vi "TestModeUpdate.vi"(8 "error in (no error)":errorcluster, 11 "Update?":bool) -> (0 "error out":errorcluster, 3 "conf'":T1={"Test Mode"=enum."6.3.2 저온 작동/방치 시험", "ON time[ms]"=500.0, "OFF time[ms]"=10000.0, "1. 작동시간[분]"=10000.0, "2. 미작동시간[분]"=10000.0, "3. 작동시간[분]"=10000.0, "level[V]"=12.0, "duty"=20.0, "Freq"=1.0, "Voltage+[V]"=20.0, "Voltage-[V]"=-20.0, "Current+[A]"=5.0, "Current-[A]"=-5.0, "출력전압[V]"=0.0, "출력전류[A]"=0.0, "OVP Level"=0.0, "OCP Level"=0.0, "Time Div"=0, "Record Len"=4, "방전 기준[V]"=0.0, "Repeate (Each Ch)"=1, "Cycle[N]"=1, "작동간격[분]"=10000.0, "TrigPos[%]"=0.0, "시험시간[분]"=10000.0} {"시험시간[분]" min=1.0; "작동간격[분]" min=1.0; "3. 작동시간[분]" min=1.0; "2. 미작동시간[분]" min=1.0; "1. 작동시간[분]" min=1.0; "Time Div" items=["10m", "20ms", "50ms", "100ms", "200ms", "500ms", "1s", "2s", "5s", "10s", "20s", "30s", "1min", "2min", "5min"]; "OFF time[ms]" min=10000.0 max=1000000.0; "Current-[A]" min=-20.0 max=20.0 step=0.001; "Voltage-[V]" min=-115.0 max=115.0 step=0.01; "Current+[A]" min=0.0 max=60.0 step=0.01; "Voltage+[V]" min=0.0 max=120.0 step=0.1; "OCP Level" format="%#_13g"; "OVP Level" format="%#_13g"; "Record Len" items=["10k", "25k", "50k", "100k", "250k", "500k", "1M", "2.5M", "5M", "10M", "25M", "50M", "100M", "250M", "500M", "1G", "2G", "4G", "5G", "10G", "20G", "50G"]; "ON time[ms]" min=50.0 max=2000000.0})   [LabVIEW 2019]
uses:
  Durability/Capacitor/cap_config.ctl
  _ctrl/rw.ctl
  Durability/common/Global 1.vi
panel:
  out "Array":string[](array[string])
  # "제어단 전압"
  # "출력단 전원"
  # "DL950"
  # "Discharge"
  # "Test Cycle"
  # "작동 설정"
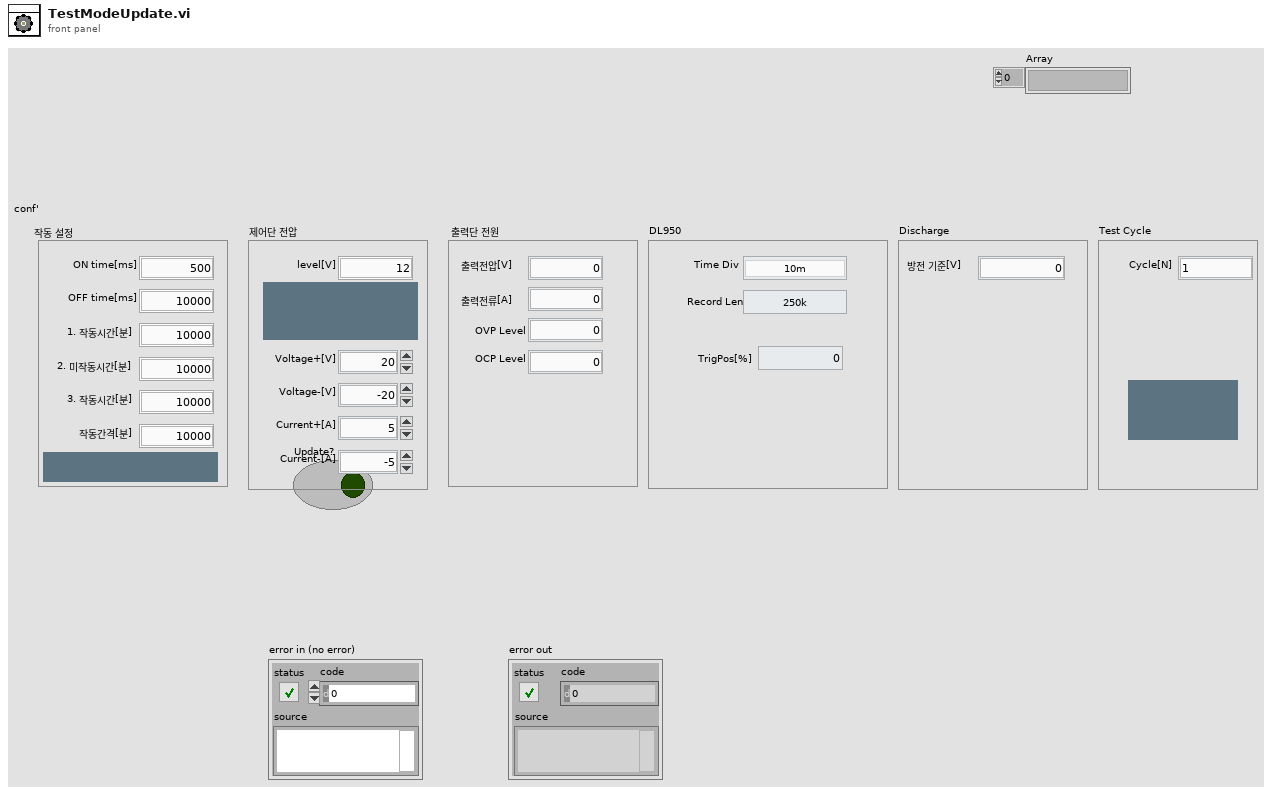
[diagram p1: front panel]
types:
  T1 = typedef "cap_config.ctl" = cluster{"Test Mode":T2, "ON time[ms]":dbl, "OFF time[ms]":dbl, "1. 작동시간[분]":dbl, "2. 미작동시간[분]":dbl, "3. 작동시간[분]":dbl, "level[V]":dbl, "duty":dbl, "Freq":dbl, "Voltage+[V]":dbl, "Voltage-[V]":dbl, "Current+[A]":dbl, "Current-[A]":dbl, "출력전압[V]":dbl, "출력전류[A]":dbl, "OVP Level":dbl, "OCP Level":dbl, "Time Div":u16, "Record Len":i32, "방전 기준[V]":dbl, "Repeate (Each Ch)":u32, "Cycle[N]":u32, "작동간격[분]":dbl, "TrigPos[%]":dbl, "시험시간[분]":dbl}
  T2 = typedef "시험모드선택.ctl" = enum16{"6.3.1 온도방치 시험", "6.3.2 저온 작동/방치 시험", "6.3.3 고온 작동/방치 시험", "6.3.4 온도 싸이클 시험", "6.3.6 온습도 싸이클 시험", "6.3.7 고온고습 방치", "6.3.8 결로 시험", "6.3.9 빙결시험", "6.3.10 공진", "6.3.11.1 작동가진", "6.3.11.2 비작동 가진 ", "6.3.12 충격시험"}
  T3 = typedef "rw.ctl" = enum16{"read", "write"}
  T4 = typedef "ref_all.ctl" = cluster{"BP4610 Config":refnum<vi>, "DSP1950 Config":refnum<vi>, "2470-config":refnum<vi>, "cDAQ 9269 AO config":refnum<vi>, "cDAQ 9221 Config":refnum<vi>, "cDAQ-9467 Config":refnum<vi>, "Waveform":refnum<vi>, "DL950 wfm":refnum<vi>, "AI Graph":refnum<vi>, "AO_Wave-config":refnum<vi>, "DL950 items":refnum<vi>, "Volt":refnum<vi>, "Current":refnum<vi>, "AO_Level":refnum<vi>, "RC-Test Judgement ":refnum<vi>, "Log path":refnum<vi>, "시험명":refnum<vi>, "file renew[Hr]":refnum<vi>, "Breakdown-Spec":refnum<vi>, "paste":refnum<vi>, "copy":refnum<vi>, "DL950_config":refnum<vi>, "종료시간":refnum<vi>, "경과시간":refnum<vi>, "Apply":refnum<vi>, "DSP Config LV ":refnum<vi>, "Testconfig":refnum<vi>}
  T5 = typedef "Test Mode.ctl" = enum32{"저항부하", "캐패시터부하", "B수명 - 1", "B수명 - 2", "B수명 - 3", "저전압모드 동작검사", "저전압모드 접촉저항", "고전압모드 동작검사"}
  T6 = enum32{"6.3.2 저온 작동/방치 시험", "6.3.3 고온 작동/방치 시험", "6.3.4 온도 싸이클 시험", "6.3.6 온습도 싸이클 시험", "6.3.8 결로 시험", "6.3.9 빙결 시험"}
  T7 = enum8{"Enabled", "Disabled", "Disabled and Grayed Out"}[]
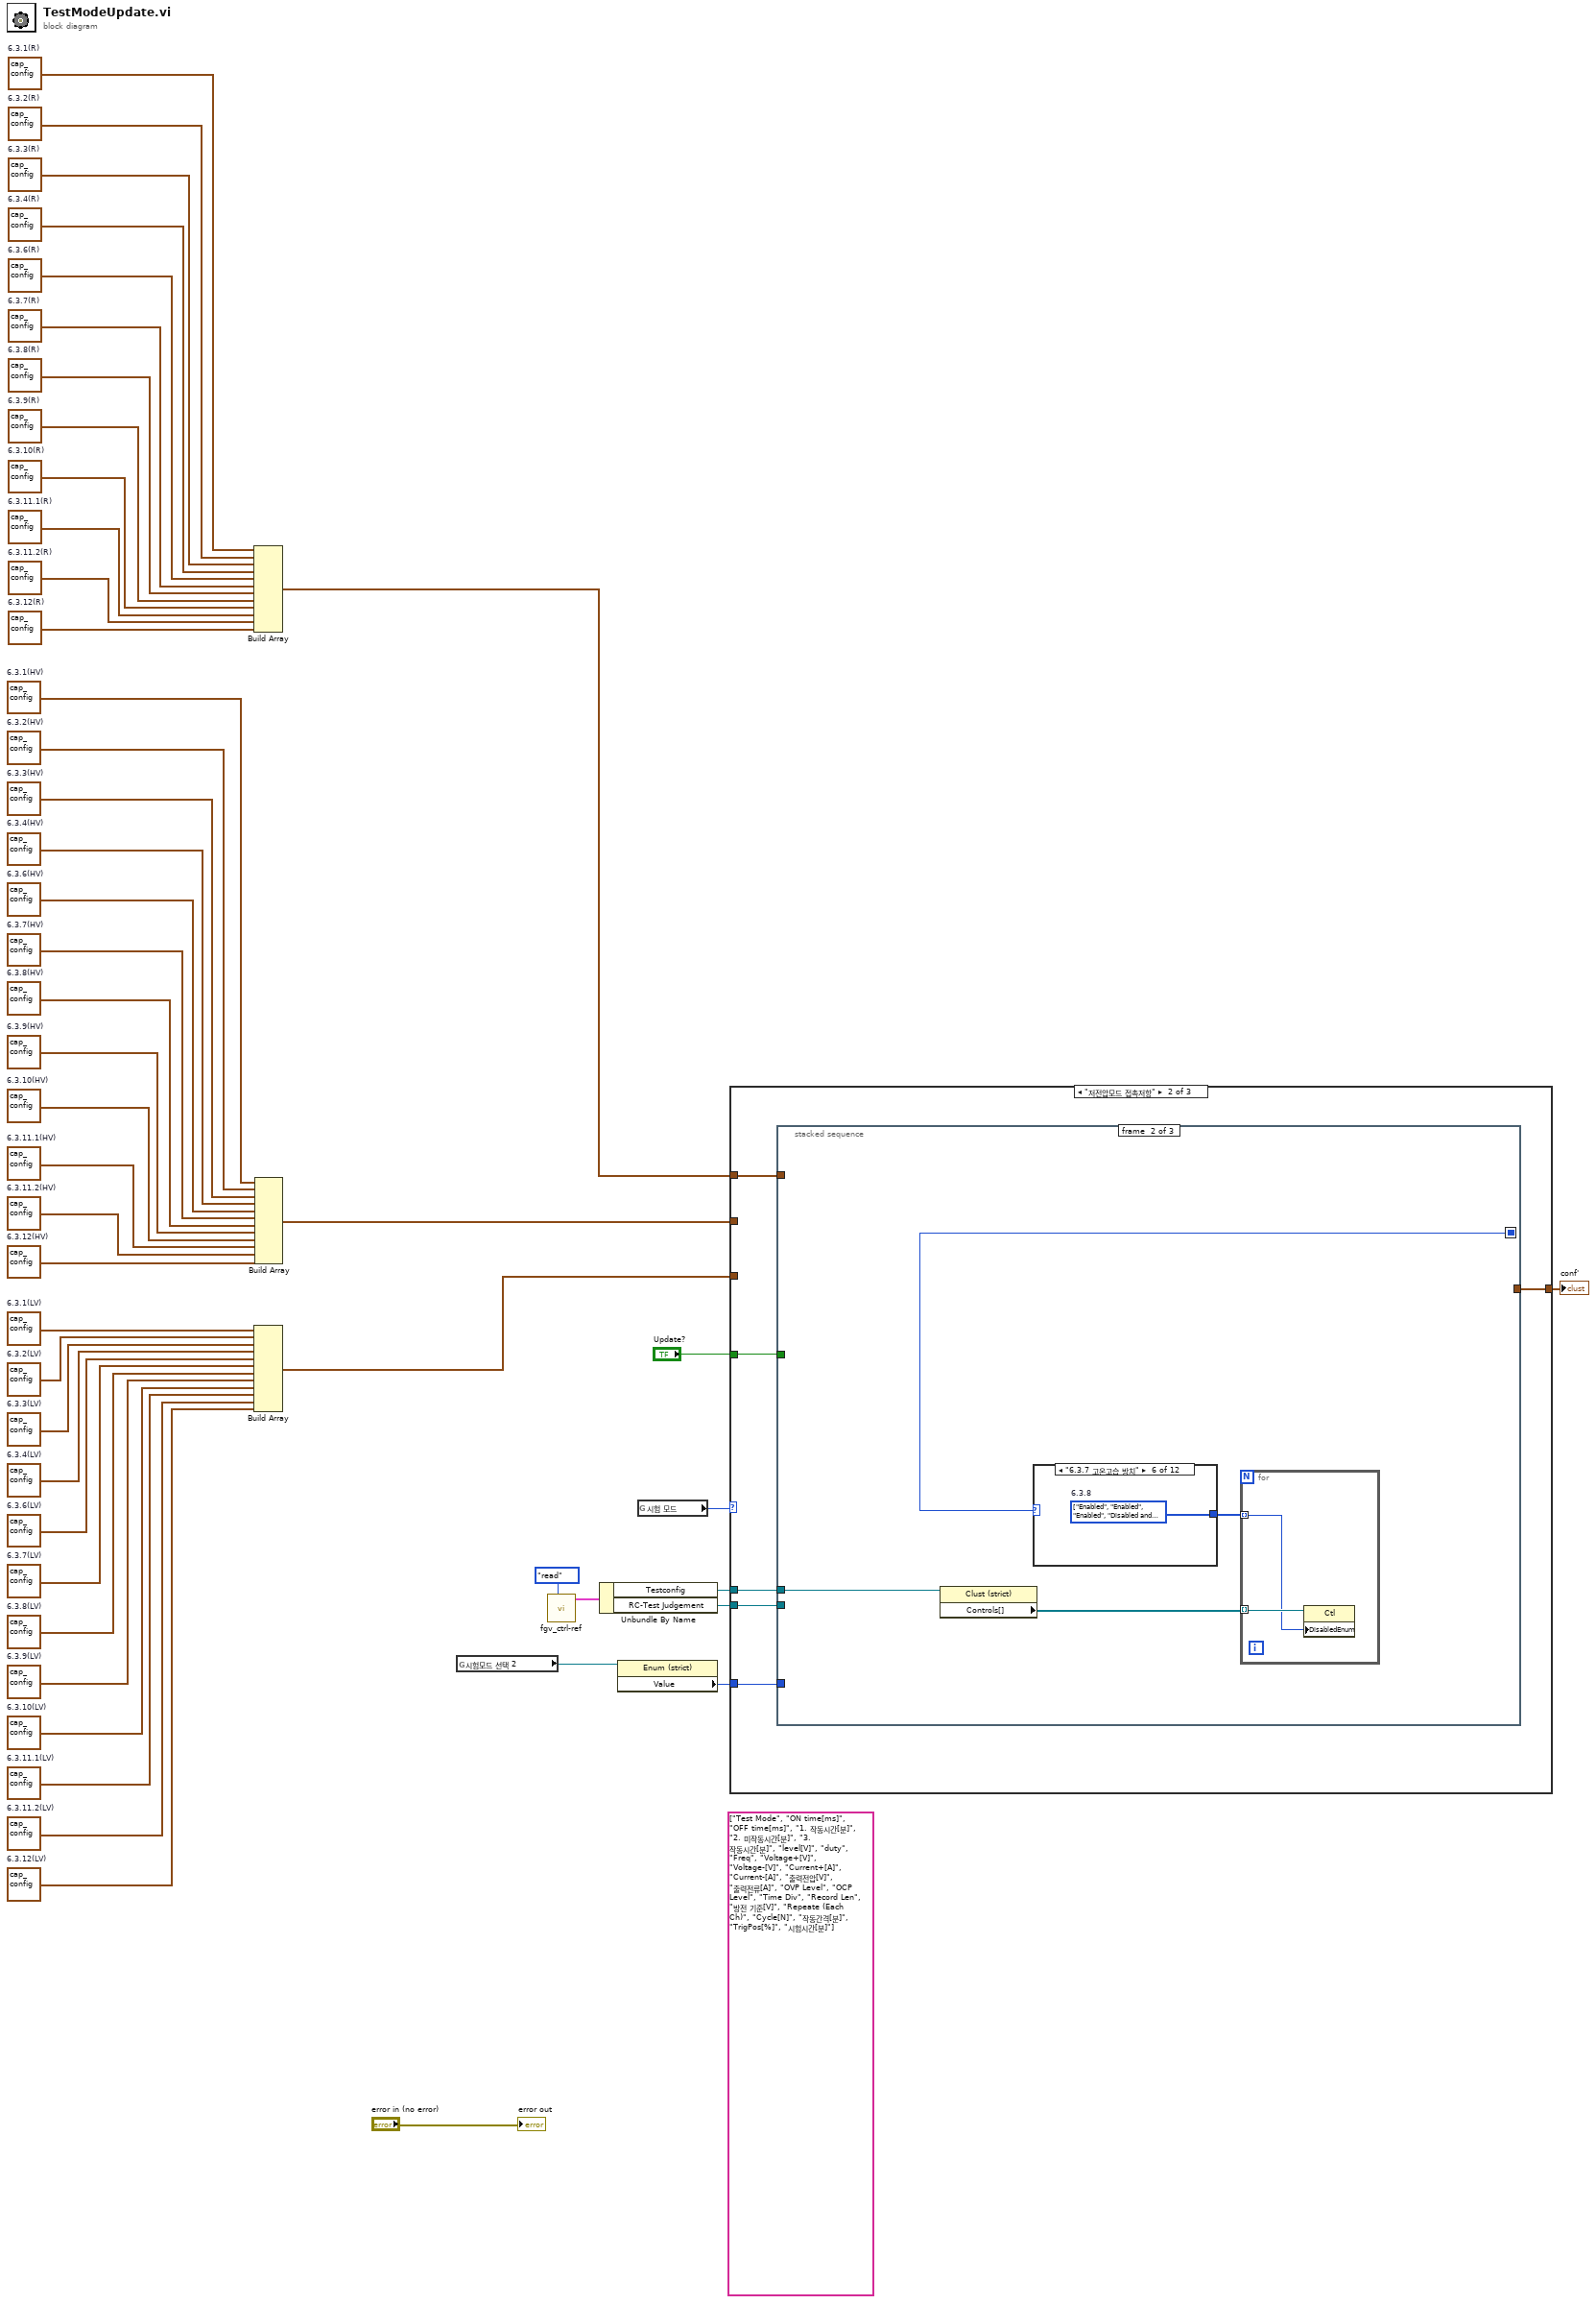
[diagram p0: block diagram]
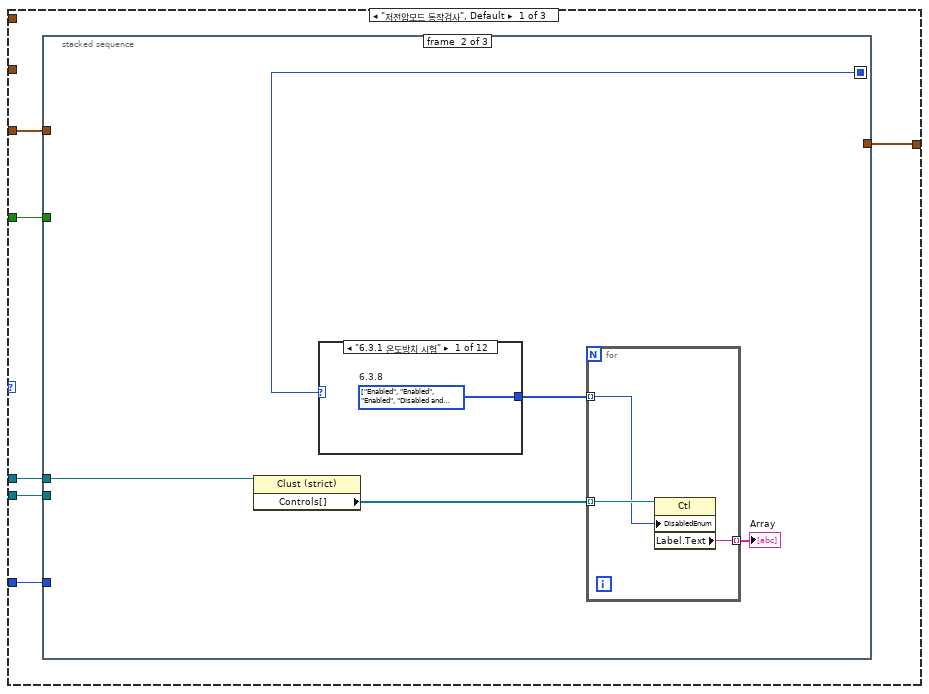
[diagram p2: hidden frame]
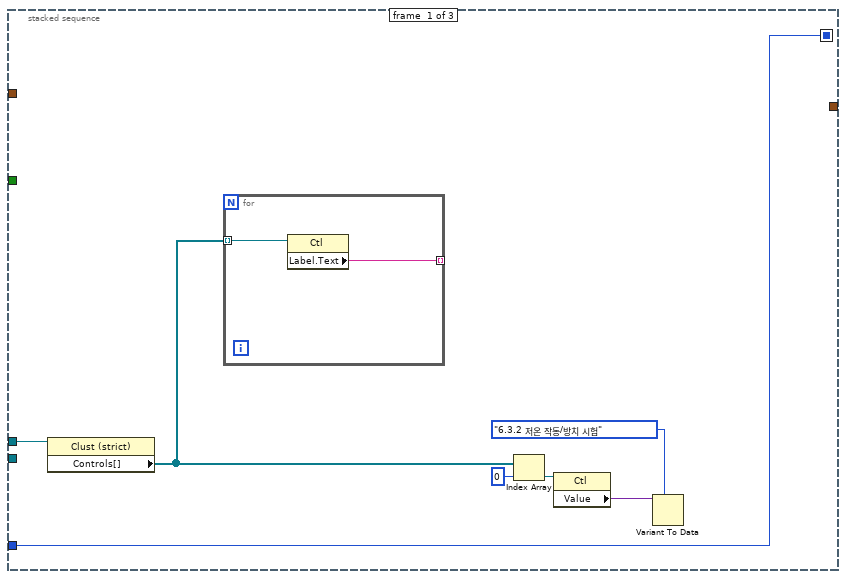
[diagram p3: hidden frame]
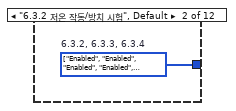
[diagram p4: hidden frame]
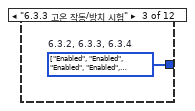
[diagram p5: hidden frame]
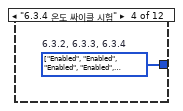
[diagram p6: hidden frame]
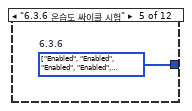
[diagram p7: hidden frame]
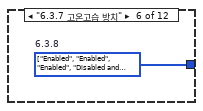
[diagram p8: hidden frame]
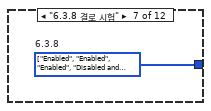
[diagram p9: hidden frame]
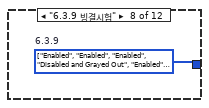
[diagram p10: hidden frame]
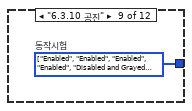
[diagram p11: hidden frame]
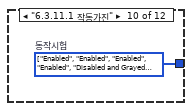
[diagram p12: hidden frame]
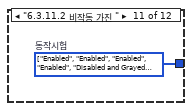
[diagram p13: hidden frame]
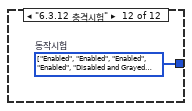
[diagram p14: hidden frame]
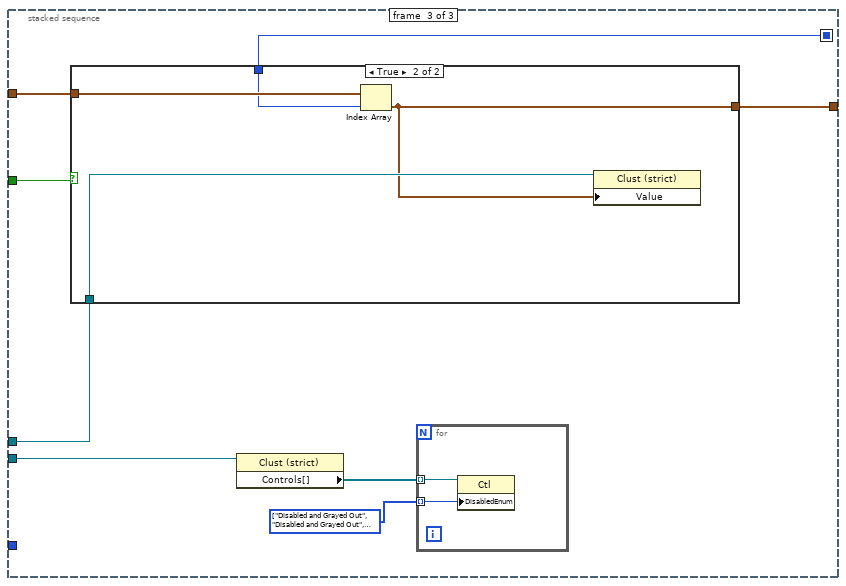
[diagram p15: hidden frame]
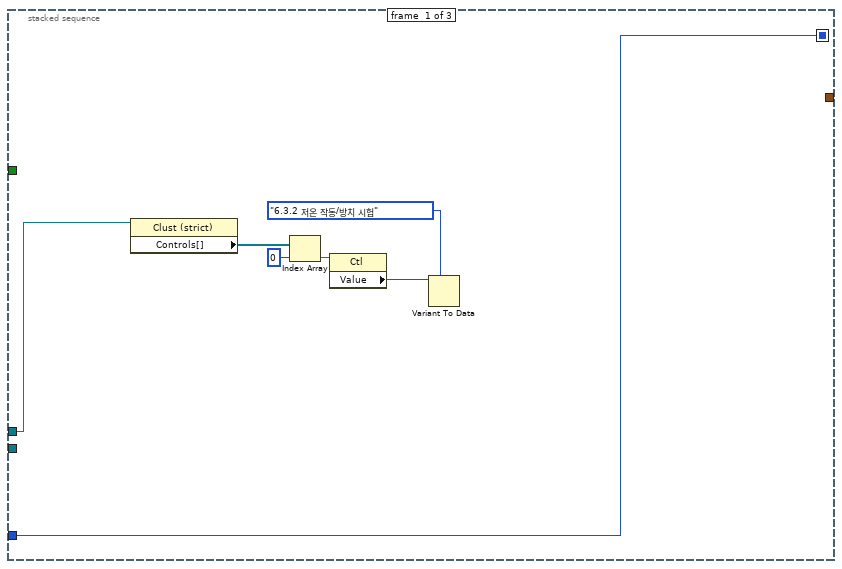
[diagram p17: hidden frame]
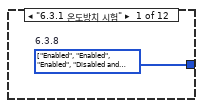
[diagram p18: hidden frame]
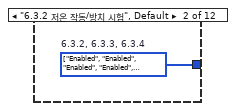
[diagram p19: hidden frame]
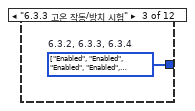
[diagram p20: hidden frame]
diagram:
  (unwired) string[] ["Test Mode", "ON time[ms]", "OFF time[ms]", "1. 작동시간[분]", "2. 미작동시간[분]", "3. 작동시간[분]", "level[V]", "duty", "Freq", "Voltage+[V]", "Voltage-[V]", "Current+[A]", "Current-[A]", "출력전압[V]", "출력전류[A]", "OVP Level", "OCP Level", "Time Div", "Record Len", "방전 기준[V]", "Repeate (Each Ch)", "Cycle[N]", "작동간격[분]", "TrigPos[%]", "시험시간[분]"] ("Array")
  w2 = T1 {"Test Mode"=enum."6.3.11.2 비작동 가진 ", "ON time[ms]"=200.0, "OFF time[ms]"=10000.0, "1. 작동시간[분]"=5.0, "2. 미작동시간[분]"=0.0, "3. 작동시간[분]"=0.0, "level[V]"=12.0, "duty"=100.0, "Freq"=1.0, "Voltage+[V]"=20.0, "Voltage-[V]"=-20.0, "Current+[A]"=5.0, "Current-[A]"=-5.0, "출력전압[V]"=12.0, "출력전류[A]"=2.0, "OVP Level"=20.0, "OCP Level"=5.0, "Time Div"=2, "Record Len"=5, "방전 기준[V]"=0.0, "Repeate (Each Ch)"=1, "Cycle[N]"=1, "작동간격[분]"=0.0, "TrigPos[%]"=10.0, "시험시간[분]"=0.0}  # 6.3.11.2(LV)
  w4 = T1 {"Test Mode"=enum."6.3.10 공진", "ON time[ms]"=200.0, "OFF time[ms]"=10000.0, "1. 작동시간[분]"=20.0, "2. 미작동시간[분]"=0.0, "3. 작동시간[분]"=0.0, "level[V]"=12.0, "duty"=100.0, "Freq"=1.0, "Voltage+[V]"=20.0, "Voltage-[V]"=-20.0, "Current+[A]"=5.0, "Current-[A]"=-5.0, "출력전압[V]"=12.0, "출력전류[A]"=2.0, "OVP Level"=20.0, "OCP Level"=5.0, "Time Div"=2, "Record Len"=5, "방전 기준[V]"=0.0, "Repeate (Each Ch)"=1, "Cycle[N]"=1, "작동간격[분]"=0.0, "TrigPos[%]"=10.0, "시험시간[분]"=0.0}  # 6.3.10(LV)
  w6 = T1 {"Test Mode"=enum."6.3.11.2 비작동 가진 ", "ON time[ms]"=200.0, "OFF time[ms]"=10000.0, "1. 작동시간[분]"=5.0, "2. 미작동시간[분]"=0.0, "3. 작동시간[분]"=0.0, "level[V]"=12.0, "duty"=100.0, "Freq"=1.0, "Voltage+[V]"=20.0, "Voltage-[V]"=-20.0, "Current+[A]"=5.0, "Current-[A]"=-5.0, "출력전압[V]"=450.0, "출력전류[A]"=30.0, "OVP Level"=1000.0, "OCP Level"=50.0, "Time Div"=2, "Record Len"=5, "방전 기준[V]"=1.0, "Repeate (Each Ch)"=1, "Cycle[N]"=1, "작동간격[분]"=0.0, "TrigPos[%]"=10.0, "시험시간[분]"=0.0}  # 6.3.11.2(HV)
  w8 = T1 {"Test Mode"=enum."6.3.10 공진", "ON time[ms]"=200.0, "OFF time[ms]"=10000.0, "1. 작동시간[분]"=20.0, "2. 미작동시간[분]"=0.0, "3. 작동시간[분]"=0.0, "level[V]"=12.0, "duty"=100.0, "Freq"=1.0, "Voltage+[V]"=20.0, "Voltage-[V]"=-20.0, "Current+[A]"=5.0, "Current-[A]"=-5.0, "출력전압[V]"=450.0, "출력전류[A]"=30.0, "OVP Level"=1000.0, "OCP Level"=50.0, "Time Div"=2, "Record Len"=5, "방전 기준[V]"=1.0, "Repeate (Each Ch)"=1, "Cycle[N]"=1, "작동간격[분]"=0.0, "TrigPos[%]"=10.0, "시험시간[분]"=0.0}  # 6.3.10(HV)
  w12 = T1 {"Test Mode"=enum."6.3.10 공진", "ON time[ms]"=200.0, "OFF time[ms]"=10000.0, "1. 작동시간[분]"=20.0, "2. 미작동시간[분]"=0.0, "3. 작동시간[분]"=0.0, "level[V]"=12.0, "duty"=100.0, "Freq"=1.0, "Voltage+[V]"=20.0, "Voltage-[V]"=-20.0, "Current+[A]"=5.0, "Current-[A]"=-5.0, "출력전압[V]"=12.0, "출력전류[A]"=1.0, "OVP Level"=20.0, "OCP Level"=5.0, "Time Div"=2, "Record Len"=5, "방전 기준[V]"=0.0, "Repeate (Each Ch)"=1, "Cycle[N]"=1, "작동간격[분]"=1.0, "TrigPos[%]"=10.0, "시험시간[분]"=1.0}  # 6.3.10(R)
  w10 = T1 {"Test Mode"=enum."6.3.11.2 비작동 가진 ", "ON time[ms]"=200.0, "OFF time[ms]"=10000.0, "1. 작동시간[분]"=5.0, "2. 미작동시간[분]"=0.0, "3. 작동시간[분]"=0.0, "level[V]"=12.0, "duty"=100.0, "Freq"=1.0, "Voltage+[V]"=20.0, "Voltage-[V]"=-20.0, "Current+[A]"=5.0, "Current-[A]"=-5.0, "출력전압[V]"=12.0, "출력전류[A]"=1.0, "OVP Level"=20.0, "OCP Level"=5.0, "Time Div"=2, "Record Len"=5, "방전 기준[V]"=0.0, "Repeate (Each Ch)"=1, "Cycle[N]"=1, "작동간격[분]"=1.0, "TrigPos[%]"=10.0, "시험시간[분]"=1.0}  # 6.3.11.2(R)
  w30 = T1 {"Test Mode"=enum."6.3.8 결로 시험", "ON time[ms]"=200.0, "OFF time[ms]"=10000.0, "1. 작동시간[분]"=1.0, "2. 미작동시간[분]"=120.0, "3. 작동시간[분]"=60.0, "level[V]"=12.0, "duty"=100.0, "Freq"=1.0, "Voltage+[V]"=20.0, "Voltage-[V]"=-20.0, "Current+[A]"=5.0, "Current-[A]"=-5.0, "출력전압[V]"=12.0, "출력전류[A]"=1.0, "OVP Level"=20.0, "OCP Level"=5.0, "Time Div"=2, "Record Len"=5, "방전 기준[V]"=0.0, "Repeate (Each Ch)"=1, "Cycle[N]"=2, "작동간격[분]"=10.0, "TrigPos[%]"=10.0, "시험시간[분]"=60.0}  # 6.3.8(R)
  w3 = T1 {"Test Mode"=enum."6.3.11.1 작동가진", "ON time[ms]"=200.0, "OFF time[ms]"=10000.0, "1. 작동시간[분]"=1440.0, "2. 미작동시간[분]"=0.0, "3. 작동시간[분]"=0.0, "level[V]"=12.0, "duty"=100.0, "Freq"=1.0, "Voltage+[V]"=20.0, "Voltage-[V]"=-20.0, "Current+[A]"=5.0, "Current-[A]"=-5.0, "출력전압[V]"=12.0, "출력전류[A]"=2.0, "OVP Level"=20.0, "OCP Level"=5.0, "Time Div"=2, "Record Len"=5, "방전 기준[V]"=0.0, "Repeate (Each Ch)"=1, "Cycle[N]"=1, "작동간격[분]"=0.0, "TrigPos[%]"=10.0, "시험시간[분]"=0.0}  # 6.3.11.1(LV)
  w15 = T1 {"Test Mode"=enum."6.3.7 고온고습 방치", "ON time[ms]"=200.0, "OFF time[ms]"=10000.0, "1. 작동시간[분]"=0.0, "2. 미작동시간[분]"=10080.0, "3. 작동시간[분]"=10080.0, "level[V]"=12.0, "duty"=100.0, "Freq"=1.0, "Voltage+[V]"=20.0, "Voltage-[V]"=-20.0, "Current+[A]"=5.0, "Current-[A]"=-5.0, "출력전압[V]"=12.0, "출력전류[A]"=2.0, "OVP Level"=20.0, "OCP Level"=5.0, "Time Div"=2, "Record Len"=5, "방전 기준[V]"=0.0, "Repeate (Each Ch)"=1, "Cycle[N]"=1, "작동간격[분]"=0.0, "TrigPos[%]"=10.0, "시험시간[분]"=0.0}  # 6.3.7(LV)
  w20 = T1 {"Test Mode"=enum."6.3.1 온도방치 시험", "ON time[ms]"=200.0, "OFF time[ms]"=10000.0, "1. 작동시간[분]"=0.0, "2. 미작동시간[분]"=720.0, "3. 작동시간[분]"=720.0, "level[V]"=12.0, "duty"=100.0, "Freq"=1.0, "Voltage+[V]"=20.0, "Voltage-[V]"=-20.0, "Current+[A]"=5.0, "Current-[A]"=-5.0, "출력전압[V]"=12.0, "출력전류[A]"=2.0, "OVP Level"=20.0, "OCP Level"=5.0, "Time Div"=2, "Record Len"=5, "방전 기준[V]"=0.0, "Repeate (Each Ch)"=1, "Cycle[N]"=1, "작동간격[분]"=0.0, "TrigPos[%]"=10.0, "시험시간[분]"=0.0}  # 6.3.1(LV)
  w7 = T1 {"Test Mode"=enum."6.3.11.1 작동가진", "ON time[ms]"=200.0, "OFF time[ms]"=10000.0, "1. 작동시간[분]"=1440.0, "2. 미작동시간[분]"=0.0, "3. 작동시간[분]"=0.0, "level[V]"=12.0, "duty"=100.0, "Freq"=1.0, "Voltage+[V]"=20.0, "Voltage-[V]"=-20.0, "Current+[A]"=5.0, "Current-[A]"=-5.0, "출력전압[V]"=450.0, "출력전류[A]"=30.0, "OVP Level"=1000.0, "OCP Level"=50.0, "Time Div"=2, "Record Len"=5, "방전 기준[V]"=1.0, "Repeate (Each Ch)"=1, "Cycle[N]"=1, "작동간격[분]"=0.0, "TrigPos[%]"=10.0, "시험시간[분]"=0.0}  # 6.3.11.1(HV)
  w23 = T1 {"Test Mode"=enum."6.3.7 고온고습 방치", "ON time[ms]"=200.0, "OFF time[ms]"=10000.0, "1. 작동시간[분]"=0.0, "2. 미작동시간[분]"=10080.0, "3. 작동시간[분]"=10080.0, "level[V]"=12.0, "duty"=100.0, "Freq"=1.0, "Voltage+[V]"=20.0, "Voltage-[V]"=-20.0, "Current+[A]"=5.0, "Current-[A]"=-5.0, "출력전압[V]"=450.0, "출력전류[A]"=30.0, "OVP Level"=1000.0, "OCP Level"=50.0, "Time Div"=2, "Record Len"=5, "방전 기준[V]"=1.0, "Repeate (Each Ch)"=1, "Cycle[N]"=1, "작동간격[분]"=0.0, "TrigPos[%]"=10.0, "시험시간[분]"=0.0}  # 6.3.7(HV)
  w28 = T1 {"Test Mode"=enum."6.3.1 온도방치 시험", "ON time[ms]"=200.0, "OFF time[ms]"=10000.0, "1. 작동시간[분]"=0.0, "2. 미작동시간[분]"=720.0, "3. 작동시간[분]"=720.0, "level[V]"=12.0, "duty"=100.0, "Freq"=1.0, "Voltage+[V]"=20.0, "Voltage-[V]"=-20.0, "Current+[A]"=5.0, "Current-[A]"=-5.0, "출력전압[V]"=450.0, "출력전류[A]"=30.0, "OVP Level"=1000.0, "OCP Level"=50.0, "Time Div"=2, "Record Len"=5, "방전 기준[V]"=1.0, "Repeate (Each Ch)"=1, "Cycle[N]"=1, "작동간격[분]"=0.0, "TrigPos[%]"=10.0, "시험시간[분]"=0.0}  # 6.3.1(HV)
  w9 = T1 {"Test Mode"=enum."6.3.12 충격시험", "ON time[ms]"=200.0, "OFF time[ms]"=10000.0, "1. 작동시간[분]"=10.0, "2. 미작동시간[분]"=0.0, "3. 작동시간[분]"=0.0, "level[V]"=12.0, "duty"=100.0, "Freq"=1.0, "Voltage+[V]"=20.0, "Voltage-[V]"=-20.0, "Current+[A]"=5.0, "Current-[A]"=-5.0, "출력전압[V]"=12.0, "출력전류[A]"=1.0, "OVP Level"=20.0, "OCP Level"=5.0, "Time Div"=2, "Record Len"=5, "방전 기준[V]"=0.0, "Repeate (Each Ch)"=1, "Cycle[N]"=1, "작동간격[분]"=1.0, "TrigPos[%]"=10.0, "시험시간[분]"=1.0}  # 6.3.12(R)
  w11 = T1 {"Test Mode"=enum."6.3.11.1 작동가진", "ON time[ms]"=200.0, "OFF time[ms]"=10000.0, "1. 작동시간[분]"=1440.0, "2. 미작동시간[분]"=0.0, "3. 작동시간[분]"=0.0, "level[V]"=12.0, "duty"=100.0, "Freq"=1.0, "Voltage+[V]"=20.0, "Voltage-[V]"=-20.0, "Current+[A]"=5.0, "Current-[A]"=-5.0, "출력전압[V]"=12.0, "출력전류[A]"=1.0, "OVP Level"=20.0, "OCP Level"=5.0, "Time Div"=2, "Record Len"=5, "방전 기준[V]"=0.0, "Repeate (Each Ch)"=1, "Cycle[N]"=1, "작동간격[분]"=1.0, "TrigPos[%]"=10.0, "시험시간[분]"=1.0}  # 6.3.11.1(R)
  w31 = T1 {"Test Mode"=enum."6.3.7 고온고습 방치", "ON time[ms]"=200.0, "OFF time[ms]"=10000.0, "1. 작동시간[분]"=0.0, "2. 미작동시간[분]"=10080.0, "3. 작동시간[분]"=10080.0, "level[V]"=12.0, "duty"=100.0, "Freq"=1.0, "Voltage+[V]"=20.0, "Voltage-[V]"=-20.0, "Current+[A]"=5.0, "Current-[A]"=-5.0, "출력전압[V]"=12.0, "출력전류[A]"=1.0, "OVP Level"=20.0, "OCP Level"=5.0, "Time Div"=2, "Record Len"=5, "방전 기준[V]"=0.0, "Repeate (Each Ch)"=1, "Cycle[N]"=1, "작동간격[분]"=1.0, "TrigPos[%]"=10.0, "시험시간[분]"=1.0}  # 6.3.7(R)
  w36 = T1 {"Test Mode"=enum."6.3.1 온도방치 시험", "ON time[ms]"=200.0, "OFF time[ms]"=10000.0, "1. 작동시간[분]"=0.0, "2. 미작동시간[분]"=720.0, "3. 작동시간[분]"=720.0, "level[V]"=12.0, "duty"=100.0, "Freq"=1.0, "Voltage+[V]"=20.0, "Voltage-[V]"=-20.0, "Current+[A]"=5.0, "Current-[A]"=-5.0, "출력전압[V]"=12.0, "출력전류[A]"=1.0, "OVP Level"=20.0, "OCP Level"=5.0, "Time Div"=2, "Record Len"=5, "방전 기준[V]"=0.0, "Repeate (Each Ch)"=1, "Cycle[N]"=1, "작동간격[분]"=1.0, "TrigPos[%]"=10.0, "시험시간[분]"=0.0}  # 6.3.1(R)
  w5 = T1 {"Test Mode"=enum."6.3.12 충격시험", "ON time[ms]"=200.0, "OFF time[ms]"=10000.0, "1. 작동시간[분]"=10.0, "2. 미작동시간[분]"=0.0, "3. 작동시간[분]"=0.0, "level[V]"=12.0, "duty"=100.0, "Freq"=1.0, "Voltage+[V]"=20.0, "Voltage-[V]"=-20.0, "Current+[A]"=5.0, "Current-[A]"=-5.0, "출력전압[V]"=450.0, "출력전류[A]"=30.0, "OVP Level"=1000.0, "OCP Level"=50.0, "Time Div"=2, "Record Len"=5, "방전 기준[V]"=1.0, "Repeate (Each Ch)"=1, "Cycle[N]"=1, "작동간격[분]"=0.0, "TrigPos[%]"=10.0, "시험시간[분]"=0.0}  # 6.3.12(HV)
  w1 = T1 {"Test Mode"=enum."6.3.12 충격시험", "ON time[ms]"=200.0, "OFF time[ms]"=10000.0, "1. 작동시간[분]"=10.0, "2. 미작동시간[분]"=0.0, "3. 작동시간[분]"=0.0, "level[V]"=12.0, "duty"=100.0, "Freq"=1.0, "Voltage+[V]"=20.0, "Voltage-[V]"=-20.0, "Current+[A]"=5.0, "Current-[A]"=-5.0, "출력전압[V]"=12.0, "출력전류[A]"=2.0, "OVP Level"=20.0, "OCP Level"=5.0, "Time Div"=2, "Record Len"=5, "방전 기준[V]"=0.0, "Repeate (Each Ch)"=1, "Cycle[N]"=1, "작동간격[분]"=0.0, "TrigPos[%]"=10.0, "시험시간[분]"=0.0}  # 6.3.12(LV)
  w29 = T1 {"Test Mode"=enum."6.3.9 빙결시험", "ON time[ms]"=5000.0, "OFF time[ms]"=10000.0, "1. 작동시간[분]"=0.0, "2. 미작동시간[분]"=240.0, "3. 작동시간[분]"=60.0, "level[V]"=12.0, "duty"=100.0, "Freq"=1.0, "Voltage+[V]"=20.0, "Voltage-[V]"=-20.0, "Current+[A]"=5.0, "Current-[A]"=-5.0, "출력전압[V]"=12.0, "출력전류[A]"=1.0, "OVP Level"=20.0, "OCP Level"=5.0, "Time Div"=6, "Record Len"=6, "방전 기준[V]"=0.0, "Repeate (Each Ch)"=1, "Cycle[N]"=2, "작동간격[분]"=1.0, "TrigPos[%]"=42.0, "시험시간[분]"=60.0}  # 6.3.9(R)
  w32 = T1 {"Test Mode"=enum."6.3.6 온습도 싸이클 시험", "ON time[ms]"=200.0, "OFF time[ms]"=10000.0, "1. 작동시간[분]"=870.0, "2. 미작동시간[분]"=360.0, "3. 작동시간[분]"=210.0, "level[V]"=12.0, "duty"=100.0, "Freq"=1.0, "Voltage+[V]"=20.0, "Voltage-[V]"=-20.0, "Current+[A]"=5.0, "Current-[A]"=-5.0, "출력전압[V]"=12.0, "출력전류[A]"=1.0, "OVP Level"=20.0, "OCP Level"=5.0, "Time Div"=2, "Record Len"=5, "방전 기준[V]"=0.0, "Repeate (Each Ch)"=1, "Cycle[N]"=10, "작동간격[분]"=1.0, "TrigPos[%]"=10.0, "시험시간[분]"=1.0}  # 6.3.6(R)
  w33 = T1 {"Test Mode"=enum."6.3.4 온도 싸이클 시험", "ON time[ms]"=200.0, "OFF time[ms]"=10000.0, "1. 작동시간[분]"=240.0, "2. 미작동시간[분]"=240.0, "3. 작동시간[분]"=0.0, "level[V]"=12.0, "duty"=100.0, "Freq"=1.0, "Voltage+[V]"=20.0, "Voltage-[V]"=-20.0, "Current+[A]"=5.0, "Current-[A]"=-5.0, "출력전압[V]"=12.0, "출력전류[A]"=1.0, "OVP Level"=20.0, "OCP Level"=5.0, "Time Div"=2, "Record Len"=5, "방전 기준[V]"=0.0, "Repeate (Each Ch)"=1, "Cycle[N]"=60, "작동간격[분]"=1.0, "TrigPos[%]"=10.0, "시험시간[분]"=1.0}  # 6.3.4(R)
  w34 = T1 {"Test Mode"=enum."6.3.3 고온 작동/방치 시험", "ON time[ms]"=200.0, "OFF time[ms]"=10000.0, "1. 작동시간[분]"=10.0, "2. 미작동시간[분]"=50.0, "3. 작동시간[분]"=0.0, "level[V]"=12.0, "duty"=100.0, "Freq"=1.0, "Voltage+[V]"=20.0, "Voltage-[V]"=-20.0, "Current+[A]"=5.0, "Current-[A]"=-5.0, "출력전압[V]"=12.0, "출력전류[A]"=1.0, "OVP Level"=20.0, "OCP Level"=5.0, "Time Div"=2, "Record Len"=5, "방전 기준[V]"=0.0, "Repeate (Each Ch)"=1, "Cycle[N]"=168, "작동간격[분]"=1.0, "TrigPos[%]"=10.0, "시험시간[분]"=1.0}  # 6.3.3(R)
  w35 = T1 {"Test Mode"=enum."6.3.2 저온 작동/방치 시험", "ON time[ms]"=200.0, "OFF time[ms]"=10000.0, "1. 작동시간[분]"=10.0, "2. 미작동시간[분]"=50.0, "3. 작동시간[분]"=0.0, "level[V]"=12.0, "duty"=100.0, "Freq"=1.0, "Voltage+[V]"=20.0, "Voltage-[V]"=-20.0, "Current+[A]"=5.0, "Current-[A]"=-5.0, "출력전압[V]"=12.0, "출력전류[A]"=1.0, "OVP Level"=20.0, "OCP Level"=5.0, "Time Div"=2, "Record Len"=5, "방전 기준[V]"=0.0, "Repeate (Each Ch)"=1, "Cycle[N]"=168, "작동간격[분]"=1.0, "TrigPos[%]"=10.0, "시험시간[분]"=1.0}  # 6.3.2(R)
  w21 = T1 {"Test Mode"=enum."6.3.9 빙결시험", "ON time[ms]"=5000.0, "OFF time[ms]"=10000.0, "1. 작동시간[분]"=0.0, "2. 미작동시간[분]"=240.0, "3. 작동시간[분]"=60.0, "level[V]"=12.0, "duty"=100.0, "Freq"=1.0, "Voltage+[V]"=20.0, "Voltage-[V]"=-20.0, "Current+[A]"=5.0, "Current-[A]"=-5.0, "출력전압[V]"=450.0, "출력전류[A]"=30.0, "OVP Level"=1000.0, "OCP Level"=50.0, "Time Div"=6, "Record Len"=6, "방전 기준[V]"=1.0, "Repeate (Each Ch)"=1, "Cycle[N]"=2, "작동간격[분]"=1.0, "TrigPos[%]"=42.0, "시험시간[분]"=60.0}  # 6.3.9(HV)
  w22 = T1 {"Test Mode"=enum."6.3.8 결로 시험", "ON time[ms]"=200.0, "OFF time[ms]"=10000.0, "1. 작동시간[분]"=0.0, "2. 미작동시간[분]"=120.0, "3. 작동시간[분]"=60.0, "level[V]"=12.0, "duty"=100.0, "Freq"=1.0, "Voltage+[V]"=20.0, "Voltage-[V]"=-20.0, "Current+[A]"=5.0, "Current-[A]"=-5.0, "출력전압[V]"=450.0, "출력전류[A]"=30.0, "OVP Level"=1000.0, "OCP Level"=50.0, "Time Div"=2, "Record Len"=5, "방전 기준[V]"=1.0, "Repeate (Each Ch)"=1, "Cycle[N]"=2, "작동간격[분]"=10.0, "TrigPos[%]"=10.0, "시험시간[분]"=60.0}  # 6.3.8(HV)
  w24 = T1 {"Test Mode"=enum."6.3.6 온습도 싸이클 시험", "ON time[ms]"=200.0, "OFF time[ms]"=10000.0, "1. 작동시간[분]"=870.0, "2. 미작동시간[분]"=360.0, "3. 작동시간[분]"=210.0, "level[V]"=12.0, "duty"=100.0, "Freq"=1.0, "Voltage+[V]"=20.0, "Voltage-[V]"=-20.0, "Current+[A]"=5.0, "Current-[A]"=-5.0, "출력전압[V]"=450.0, "출력전류[A]"=30.0, "OVP Level"=1000.0, "OCP Level"=50.0, "Time Div"=2, "Record Len"=5, "방전 기준[V]"=1.0, "Repeate (Each Ch)"=1, "Cycle[N]"=10, "작동간격[분]"=1.0, "TrigPos[%]"=10.0, "시험시간[분]"=1.0}  # 6.3.6(HV)
  w25 = T1 {"Test Mode"=enum."6.3.4 온도 싸이클 시험", "ON time[ms]"=200.0, "OFF time[ms]"=10000.0, "1. 작동시간[분]"=240.0, "2. 미작동시간[분]"=240.0, "3. 작동시간[분]"=0.0, "level[V]"=12.0, "duty"=100.0, "Freq"=1.0, "Voltage+[V]"=20.0, "Voltage-[V]"=-20.0, "Current+[A]"=5.0, "Current-[A]"=-5.0, "출력전압[V]"=450.0, "출력전류[A]"=30.0, "OVP Level"=1000.0, "OCP Level"=50.0, "Time Div"=2, "Record Len"=5, "방전 기준[V]"=1.0, "Repeate (Each Ch)"=1, "Cycle[N]"=60, "작동간격[분]"=1.0, "TrigPos[%]"=10.0, "시험시간[분]"=1.0}  # 6.3.4(HV)
  w26 = T1 {"Test Mode"=enum."6.3.3 고온 작동/방치 시험", "ON time[ms]"=200.0, "OFF time[ms]"=10000.0, "1. 작동시간[분]"=10.0, "2. 미작동시간[분]"=50.0, "3. 작동시간[분]"=0.0, "level[V]"=12.0, "duty"=100.0, "Freq"=1.0, "Voltage+[V]"=20.0, "Voltage-[V]"=-20.0, "Current+[A]"=5.0, "Current-[A]"=-5.0, "출력전압[V]"=450.0, "출력전류[A]"=30.0, "OVP Level"=1000.0, "OCP Level"=50.0, "Time Div"=2, "Record Len"=5, "방전 기준[V]"=1.0, "Repeate (Each Ch)"=1, "Cycle[N]"=168, "작동간격[분]"=1.0, "TrigPos[%]"=10.0, "시험시간[분]"=1.0}  # 6.3.3(HV)
  w27 = T1 {"Test Mode"=enum."6.3.2 저온 작동/방치 시험", "ON time[ms]"=200.0, "OFF time[ms]"=10000.0, "1. 작동시간[분]"=10.0, "2. 미작동시간[분]"=50.0, "3. 작동시간[분]"=0.0, "level[V]"=12.0, "duty"=100.0, "Freq"=1.0, "Voltage+[V]"=20.0, "Voltage-[V]"=-20.0, "Current+[A]"=5.0, "Current-[A]"=-5.0, "출력전압[V]"=450.0, "출력전류[A]"=30.0, "OVP Level"=1000.0, "OCP Level"=50.0, "Time Div"=2, "Record Len"=5, "방전 기준[V]"=1.0, "Repeate (Each Ch)"=1, "Cycle[N]"=168, "작동간격[분]"=1.0, "TrigPos[%]"=10.0, "시험시간[분]"=1.0}  # 6.3.2(HV)
  w13 = T1 {"Test Mode"=enum."6.3.9 빙결시험", "ON time[ms]"=5000.0, "OFF time[ms]"=10000.0, "1. 작동시간[분]"=0.0, "2. 미작동시간[분]"=240.0, "3. 작동시간[분]"=60.0, "level[V]"=12.0, "duty"=100.0, "Freq"=1.0, "Voltage+[V]"=20.0, "Voltage-[V]"=-20.0, "Current+[A]"=5.0, "Current-[A]"=-5.0, "출력전압[V]"=12.0, "출력전류[A]"=2.0, "OVP Level"=20.0, "OCP Level"=5.0, "Time Div"=6, "Record Len"=6, "방전 기준[V]"=0.0, "Repeate (Each Ch)"=1, "Cycle[N]"=2, "작동간격[분]"=1.0, "TrigPos[%]"=42.0, "시험시간[분]"=60.0}  # 6.3.9(LV)
  w14 = T1 {"Test Mode"=enum."6.3.8 결로 시험", "ON time[ms]"=200.0, "OFF time[ms]"=10000.0, "1. 작동시간[분]"=0.0, "2. 미작동시간[분]"=120.0, "3. 작동시간[분]"=60.0, "level[V]"=12.0, "duty"=100.0, "Freq"=1.0, "Voltage+[V]"=20.0, "Voltage-[V]"=-20.0, "Current+[A]"=5.0, "Current-[A]"=-5.0, "출력전압[V]"=12.0, "출력전류[A]"=2.0, "OVP Level"=20.0, "OCP Level"=5.0, "Time Div"=2, "Record Len"=5, "방전 기준[V]"=0.0, "Repeate (Each Ch)"=1, "Cycle[N]"=2, "작동간격[분]"=10.0, "TrigPos[%]"=10.0, "시험시간[분]"=60.0}  # 6.3.8(LV)
  w16 = T1 {"Test Mode"=enum."6.3.6 온습도 싸이클 시험", "ON time[ms]"=200.0, "OFF time[ms]"=10000.0, "1. 작동시간[분]"=870.0, "2. 미작동시간[분]"=360.0, "3. 작동시간[분]"=210.0, "level[V]"=12.0, "duty"=100.0, "Freq"=1.0, "Voltage+[V]"=20.0, "Voltage-[V]"=-20.0, "Current+[A]"=5.0, "Current-[A]"=-5.0, "출력전압[V]"=12.0, "출력전류[A]"=2.0, "OVP Level"=20.0, "OCP Level"=5.0, "Time Div"=2, "Record Len"=5, "방전 기준[V]"=0.0, "Repeate (Each Ch)"=1, "Cycle[N]"=10, "작동간격[분]"=1.0, "TrigPos[%]"=10.0, "시험시간[분]"=1.0}  # 6.3.6(LV)
  w17 = T1 {"Test Mode"=enum."6.3.4 온도 싸이클 시험", "ON time[ms]"=200.0, "OFF time[ms]"=10000.0, "1. 작동시간[분]"=240.0, "2. 미작동시간[분]"=240.0, "3. 작동시간[분]"=0.0, "level[V]"=12.0, "duty"=100.0, "Freq"=1.0, "Voltage+[V]"=20.0, "Voltage-[V]"=-20.0, "Current+[A]"=5.0, "Current-[A]"=-5.0, "출력전압[V]"=12.0, "출력전류[A]"=2.0, "OVP Level"=20.0, "OCP Level"=5.0, "Time Div"=2, "Record Len"=5, "방전 기준[V]"=0.0, "Repeate (Each Ch)"=1, "Cycle[N]"=60, "작동간격[분]"=1.0, "TrigPos[%]"=10.0, "시험시간[분]"=1.0}  # 6.3.4(LV)
  w18 = T1 {"Test Mode"=enum."6.3.3 고온 작동/방치 시험", "ON time[ms]"=200.0, "OFF time[ms]"=10000.0, "1. 작동시간[분]"=10.0, "2. 미작동시간[분]"=50.0, "3. 작동시간[분]"=0.0, "level[V]"=12.0, "duty"=100.0, "Freq"=1.0, "Voltage+[V]"=20.0, "Voltage-[V]"=-20.0, "Current+[A]"=5.0, "Current-[A]"=-5.0, "출력전압[V]"=12.0, "출력전류[A]"=2.0, "OVP Level"=20.0, "OCP Level"=5.0, "Time Div"=2, "Record Len"=5, "방전 기준[V]"=0.0, "Repeate (Each Ch)"=1, "Cycle[N]"=168, "작동간격[분]"=1.0, "TrigPos[%]"=10.0, "시험시간[분]"=1.0}  # 6.3.3(LV)
  w19 = T1 {"Test Mode"=enum."6.3.2 저온 작동/방치 시험", "ON time[ms]"=200.0, "OFF time[ms]"=10000.0, "1. 작동시간[분]"=10.0, "2. 미작동시간[분]"=50.0, "3. 작동시간[분]"=0.0, "level[V]"=12.0, "duty"=100.0, "Freq"=1.0, "Voltage+[V]"=20.0, "Voltage-[V]"=-20.0, "Current+[A]"=5.0, "Current-[A]"=-5.0, "출력전압[V]"=12.0, "출력전류[A]"=2.0, "OVP Level"=20.0, "OCP Level"=5.0, "Time Div"=2, "Record Len"=5, "방전 기준[V]"=0.0, "Repeate (Each Ch)"=1, "Cycle[N]"=168, "작동간격[분]"=1.0, "TrigPos[%]"=10.0, "시험시간[분]"=1.0}  # 6.3.2(LV)
  n1 = Build Array(w36, w35, w34, w33, w32, w31, w30, w29, w12, w11, w10, w9) -> (w40:T1[])
  n2 = Build Array(w20, w19, w18, w17, w16, w15, w14, w13, w4, w3, w2, w1) -> (w43:T1[])
  n3 = Build Array(w28, w27, w26, w25, w24, w23, w22, w21, w8, w7, w6, w5) -> (w42:T1[])
  n4 = global read "Global 1.vi" "시험모드 선택 2"() -> (w38:refnum<vi>)
  n5 = call "fgv_ctrl-ref.vi"("cmd"=rw."read") -> ("output cluster 2"=w48:T4)  [unwired: 9 in, 1 out]
  n6 = Unbundle By Name(w48) -> ("Testconfig"=w44:refnum<vi>, "RC-Test Judgement"=w46:refnum<vi>)
  n7 = property class="Enum (strict)"(reference=w38) -> ("Value"=w37:T2)  [unwired: 1 in, 2 out]
  n8 = global read "Global 1.vi" "시험 모드"() -> (w47:T5)
  n9 = case shown="\"저전압모드 접촉저항\"" w47 {
    tunnel: w44 -> [w55 w104 w149]
    tunnel: w46 -> [w54 w103 w148]
    tunnel: w43 -> [w53 _ _]
    tunnel: w42 -> [_ _ w147]
    tunnel: "Update?" -> [w52 w102 w146]
    tunnel: w40 -> [_ w101 _]
    tunnel: [w51 w100 w145] -> w39
    tunnel: w37 -> [w50 w99 w144]
    frame "저전압모드 동작검사", Default {
      n10 = stacked-sequence {
        seq-local: [w57 _ _] -> [_ w67 w88]
        tunnel: w55 -> [w58 w68 w87]
        tunnel: w54 -> [_ _ w92]
        tunnel: w53 -> [_ _ w89]
        tunnel: w52 -> [_ _ w86]
        tunnel: [_ _ w85] -> w51
        tunnel: w50 -> [w57 _ _]
        frame #0 {
          n11 = property class="Clust (strict)"(reference=w58) -> ("Controls[]"=w56:refnum<vi>[])  [unwired: 1 in, 2 out]
          n12 = for {
            tunnel: w56 -> [w64] mode=indexing
            tunnel: [w63] -> _ mode=indexing
            n13 = property class="Ctl"(reference=w64) -> ("Label.Text"=w63:string)  [unwired: 1 in, 2 out]
          }
          n14 = Index Array(array=w56, index=0) -> (element=w61:refnum<vi>)
          n15 = property class="Ctl"(reference=w61) -> ("Value"=w60:variant)  [unwired: 1 in, 2 out]
          n16 = Variant To Data(type=T6."6.3.2 저온 작동/방치 시험" ("Test Mode"), Variant=w60) -> ()  [unwired: 1 in, 2 out]
        }
        frame #1 {
          n17 = property class="Clust (strict)"(reference=w68) -> ("Controls[]"=w69:refnum<vi>[])  [unwired: 1 in, 2 out]
          n18 = case shown="\"6.3.1 온도방치 시험\"" w67 {
            tunnel: [w70 w71 w72 w73 w74 w75 w76 w77 w78 w79 w80 w81] -> w66
            frame "6.3.1 온도방치 시험" {
              w70 = T7 [enum."Enabled", enum."Enabled", enum."Enabled", enum."Disabled and Grayed Out", enum."Enabled", enum."Enabled", enum."Enabled", enum."Enabled", enum."Enabled", enum."Enabled", enum."Enabled", enum."Enabled", enum."Enabled", enum."Enabled", enum."Enabled", enum."Enabled", enum."Enabled", enum."Enabled", enum."Enabled", enum."Disabled and Grayed Out", enum."Enabled", enum."Disabled and Grayed Out", enum."Disabled and Grayed Out", enum."Enabled", enum."Enabled"] items=["Enabled", "Disabled", "Disabled and Grayed Out"]  # 6.3.8
            }
            frame "6.3.2 저온 작동/방치 시험", Default {
              w71 = T7 [enum."Enabled", enum."Enabled", enum."Enabled", enum."Enabled", enum."Enabled", enum."Disabled and Grayed Out", enum."Enabled", enum."Enabled", enum."Enabled", enum."Enabled", enum."Enabled", enum."Enabled", enum."Enabled", enum."Enabled", enum."Enabled", enum."Enabled", enum."Enabled", enum."Enabled", enum."Enabled", enum."Disabled and Grayed Out", enum."Enabled", enum."Enabled", enum."Disabled and Grayed Out", enum."Enabled", enum."Disabled and Grayed Out"] items=["Enabled", "Disabled", "Disabled and Grayed Out"]  # 6.3.2, 6.3.3, 6.3.4
            }
            frame "6.3.3 고온 작동/방치 시험" {
              w72 = T7 [enum."Enabled", enum."Enabled", enum."Enabled", enum."Enabled", enum."Enabled", enum."Disabled and Grayed Out", enum."Enabled", enum."Enabled", enum."Enabled", enum."Enabled", enum."Enabled", enum."Enabled", enum."Enabled", enum."Enabled", enum."Enabled", enum."Enabled", enum."Enabled", enum."Enabled", enum."Enabled", enum."Disabled and Grayed Out", enum."Enabled", enum."Enabled", enum."Disabled and Grayed Out", enum."Enabled", enum."Disabled and Grayed Out"] items=["Enabled", "Disabled", "Disabled and Grayed Out"]  # 6.3.2, 6.3.3, 6.3.4
            }
            frame "6.3.4 온도 싸이클 시험" {
              w73 = T7 [enum."Enabled", enum."Enabled", enum."Enabled", enum."Enabled", enum."Enabled", enum."Disabled and Grayed Out", enum."Enabled", enum."Enabled", enum."Enabled", enum."Enabled", enum."Enabled", enum."Enabled", enum."Enabled", enum."Enabled", enum."Enabled", enum."Enabled", enum."Enabled", enum."Enabled", enum."Enabled", enum."Disabled and Grayed Out", enum."Enabled", enum."Enabled", enum."Disabled and Grayed Out", enum."Enabled", enum."Disabled and Grayed Out"] items=["Enabled", "Disabled", "Disabled and Grayed Out"]  # 6.3.2, 6.3.3, 6.3.4
            }
            frame "6.3.6 온습도 싸이클 시험" {
              w74 = T7 [enum."Enabled", enum."Enabled", enum."Enabled", enum."Enabled", enum."Enabled", enum."Enabled", enum."Enabled", enum."Enabled", enum."Enabled", enum."Enabled", enum."Enabled", enum."Enabled", enum."Enabled", enum."Enabled", enum."Enabled", enum."Enabled", enum."Enabled", enum."Enabled", enum."Enabled", enum."Disabled and Grayed Out", enum."Enabled", enum."Enabled", enum."Disabled and Grayed Out", enum."Enabled", enum."Disabled and Grayed Out"] items=["Enabled", "Disabled", "Disabled and Grayed Out"]  # 6.3.6
            }
            frame "6.3.7 고온고습 방치" {
              w75 = T7 [enum."Enabled", enum."Enabled", enum."Enabled", enum."Disabled and Grayed Out", enum."Enabled", enum."Enabled", enum."Enabled", enum."Enabled", enum."Enabled", enum."Enabled", enum."Enabled", enum."Enabled", enum."Enabled", enum."Enabled", enum."Enabled", enum."Enabled", enum."Enabled", enum."Enabled", enum."Enabled", enum."Disabled and Grayed Out", enum."Enabled", enum."Disabled and Grayed Out", enum."Disabled and Grayed Out", enum."Enabled", enum."Enabled"] items=["Enabled", "Disabled", "Disabled and Grayed Out"]  # 6.3.8
            }
            frame "6.3.8 결로 시험" {
              w76 = T7 [enum."Enabled", enum."Enabled", enum."Enabled", enum."Disabled and Grayed Out", enum."Enabled", enum."Enabled", enum."Enabled", enum."Enabled", enum."Enabled", enum."Enabled", enum."Enabled", enum."Enabled", enum."Enabled", enum."Enabled", enum."Enabled", enum."Enabled", enum."Enabled", enum."Enabled", enum."Enabled", enum."Disabled and Grayed Out", enum."Enabled", enum."Enabled", enum."Enabled", enum."Enabled", enum."Enabled"] items=["Enabled", "Disabled", "Disabled and Grayed Out"]  # 6.3.8
            }
            frame "6.3.9 빙결시험" {
              w77 = T7 [enum."Enabled", enum."Enabled", enum."Enabled", enum."Disabled and Grayed Out", enum."Enabled", enum."Enabled", enum."Enabled", enum."Enabled", enum."Enabled", enum."Enabled", enum."Enabled", enum."Enabled", enum."Enabled", enum."Enabled", enum."Enabled", enum."Enabled", enum."Enabled", enum."Enabled", enum."Enabled", enum."Disabled and Grayed Out", enum."Enabled", enum."Enabled", enum."Disabled and Grayed Out", enum."Enabled", enum."Enabled"] items=["Enabled", "Disabled", "Disabled and Grayed Out"]  # 6.3.9
            }
            frame "6.3.10 공진" {
              w78 = T7 [enum."Enabled", enum."Enabled", enum."Enabled", enum."Enabled", enum."Disabled and Grayed Out", enum."Disabled and Grayed Out", enum."Enabled", enum."Enabled", enum."Enabled", enum."Enabled", enum."Enabled", enum."Enabled", enum."Enabled", enum."Enabled", enum."Enabled", enum."Enabled", enum."Enabled", enum."Enabled", enum."Enabled", enum."Disabled and Grayed Out", enum."Enabled", enum."Disabled and Grayed Out", enum."Disabled and Grayed Out", enum."Enabled", enum."Disabled and Grayed Out"] items=["Enabled", "Disabled", "Disabled and Grayed Out"]  # 동작시험
            }
            frame "6.3.11.1 작동가진" {
              w79 = T7 [enum."Enabled", enum."Enabled", enum."Enabled", enum."Enabled", enum."Disabled and Grayed Out", enum."Disabled and Grayed Out", enum."Enabled", enum."Enabled", enum."Enabled", enum."Enabled", enum."Enabled", enum."Enabled", enum."Enabled", enum."Enabled", enum."Enabled", enum."Enabled", enum."Enabled", enum."Enabled", enum."Enabled", enum."Disabled and Grayed Out", enum."Enabled", enum."Disabled and Grayed Out", enum."Disabled and Grayed Out", enum."Enabled", enum."Disabled and Grayed Out"] items=["Enabled", "Disabled", "Disabled and Grayed Out"]  # 동작시험
            }
            frame "6.3.11.2 비작동 가진 " {
              w80 = T7 [enum."Enabled", enum."Enabled", enum."Enabled", enum."Enabled", enum."Disabled and Grayed Out", enum."Disabled and Grayed Out", enum."Enabled", enum."Enabled", enum."Enabled", enum."Enabled", enum."Enabled", enum."Enabled", enum."Enabled", enum."Enabled", enum."Enabled", enum."Enabled", enum."Enabled", enum."Enabled", enum."Enabled", enum."Disabled and Grayed Out", enum."Enabled", enum."Disabled and Grayed Out", enum."Disabled and Grayed Out", enum."Enabled", enum."Disabled and Grayed Out"] items=["Enabled", "Disabled", "Disabled and Grayed Out"]  # 동작시험
            }
            frame "6.3.12 충격시험" {
              w81 = T7 [enum."Enabled", enum."Enabled", enum."Enabled", enum."Enabled", enum."Disabled and Grayed Out", enum."Disabled and Grayed Out", enum."Enabled", enum."Enabled", enum."Enabled", enum."Enabled", enum."Enabled", enum."Enabled", enum."Enabled", enum."Enabled", enum."Enabled", enum."Enabled", enum."Enabled", enum."Enabled", enum."Enabled", enum."Disabled and Grayed Out", enum."Enabled", enum."Disabled and Grayed Out", enum."Disabled and Grayed Out", enum."Enabled", enum."Disabled and Grayed Out"] items=["Enabled", "Disabled", "Disabled and Grayed Out"]  # 동작시험
            }
          }
          n19 = for {
            tunnel: w69 -> [w84] mode=indexing
            tunnel: w66 -> [w83] mode=indexing
            tunnel: [w82] -> w65 mode=indexing
            n20 = property class="Ctl"(reference=w84, "DisabledEnum"=w83) -> ("Label.Text"=w82:string)  [unwired: 1 in, 2 out]
          }
          "Array" <- w65
        }
        frame #2 {
          w90 = T7 [enum."Disabled and Grayed Out", enum."Disabled and Grayed Out", enum."Disabled and Grayed Out", enum."Disabled and Grayed Out", enum."Enabled", enum."Disabled and Grayed Out", enum."Disabled and Grayed Out", enum."Disabled and Grayed Out", enum."Disabled and Grayed Out", enum."Enabled"] items=["Enabled", "Disabled", "Disabled and Grayed Out"]
          n21 = case shown="True" w86 {
            tunnel: w89 -> [_ w96]
            tunnel: w88 -> [_ w95]
            tunnel: w87 -> [_ w94]
            tunnel: [_ w93] -> w85
            frame False {
            }
            frame True {
              n22 = Index Array(array=w96, index=w95) -> (element=w93:T1)
              n23 = property class="Clust (strict)"(reference=w94, "Value"=w93) -> ()  [unwired: 1 in, 2 out]
            }
          }
          n24 = property class="Clust (strict)"(reference=w92) -> ("Controls[]"=w91:refnum<vi>[])  [unwired: 1 in, 2 out]
          n25 = for {
            tunnel: w91 -> [w98] mode=indexing
            tunnel: w90 -> [w97] mode=indexing
            n26 = property class="Ctl"(reference=w98, "DisabledEnum"=w97) -> ()  [unwired: 1 in, 2 out]
          }
        }
      }
    }
    frame "저전압모드 접촉저항" {
      n27 = stacked-sequence {
        seq-local: [w105 _ _] -> [_ w113 w134]
        tunnel: w104 -> [w111 w115 w133]
        tunnel: w103 -> [_ _ w137]
        tunnel: w102 -> [_ _ w132]
        tunnel: w101 -> [_ _ w131]
        tunnel: [_ _ w130] -> w100
        tunnel: w99 -> [w105 _ _]
        frame #0 {
          n28 = property class="Clust (strict)"(reference=w111) -> ("Controls[]"=w108:refnum<vi>[])  [unwired: 1 in, 2 out]
          n29 = Index Array(array=w108, index=0) -> (element=w109:refnum<vi>)
          n30 = property class="Ctl"(reference=w109) -> ("Value"=w107:variant)  [unwired: 1 in, 2 out]
          n31 = Variant To Data(type=T6."6.3.2 저온 작동/방치 시험" ("Test Mode"), Variant=w107) -> ()  [unwired: 1 in, 2 out]
        }
        frame #1 {
          n32 = property class="Clust (strict)"(reference=w115) -> ("Controls[]"=w114:refnum<vi>[])  [unwired: 1 in, 2 out]
          n33 = case shown="\"6.3.7 고온고습 방치\"" w113 {
            tunnel: [w116 w117 w118 w119 w120 w121 w122 w123 w124 w125 w126 w127] -> w112
            frame "6.3.1 온도방치 시험" {
              w116 = T7 [enum."Enabled", enum."Enabled", enum."Enabled", enum."Disabled and Grayed Out", enum."Enabled", enum."Enabled", enum."Enabled", enum."Enabled", enum."Enabled", enum."Enabled", enum."Enabled", enum."Enabled", enum."Enabled", enum."Enabled", enum."Enabled", enum."Enabled", enum."Enabled", enum."Enabled", enum."Enabled", enum."Disabled and Grayed Out", enum."Enabled", enum."Disabled and Grayed Out", enum."Disabled and Grayed Out", enum."Enabled", enum."Enabled"] items=["Enabled", "Disabled", "Disabled and Grayed Out"]  # 6.3.8
            }
            frame "6.3.2 저온 작동/방치 시험", Default {
              w117 = T7 [enum."Enabled", enum."Enabled", enum."Enabled", enum."Enabled", enum."Enabled", enum."Disabled and Grayed Out", enum."Enabled", enum."Enabled", enum."Enabled", enum."Enabled", enum."Enabled", enum."Enabled", enum."Enabled", enum."Enabled", enum."Enabled", enum."Enabled", enum."Enabled", enum."Enabled", enum."Enabled", enum."Disabled and Grayed Out", enum."Enabled", enum."Enabled", enum."Disabled and Grayed Out", enum."Enabled", enum."Disabled and Grayed Out"] items=["Enabled", "Disabled", "Disabled and Grayed Out"]  # 6.3.2, 6.3.3, 6.3.4
            }
            frame "6.3.3 고온 작동/방치 시험" {
              w118 = T7 [enum."Enabled", enum."Enabled", enum."Enabled", enum."Enabled", enum."Enabled", enum."Disabled and Grayed Out", enum."Enabled", enum."Enabled", enum."Enabled", enum."Enabled", enum."Enabled", enum."Enabled", enum."Enabled", enum."Enabled", enum."Enabled", enum."Enabled", enum."Enabled", enum."Enabled", enum."Enabled", enum."Disabled and Grayed Out", enum."Enabled", enum."Enabled", enum."Disabled and Grayed Out", enum."Enabled", enum."Disabled and Grayed Out"] items=["Enabled", "Disabled", "Disabled and Grayed Out"]  # 6.3.2, 6.3.3, 6.3.4
            }
            frame "6.3.4 온도 싸이클 시험" {
              w119 = T7 [enum."Enabled", enum."Enabled", enum."Enabled", enum."Enabled", enum."Enabled", enum."Disabled and Grayed Out", enum."Enabled", enum."Enabled", enum."Enabled", enum."Enabled", enum."Enabled", enum."Enabled", enum."Enabled", enum."Enabled", enum."Enabled", enum."Enabled", enum."Enabled", enum."Enabled", enum."Enabled", enum."Disabled and Grayed Out", enum."Enabled", enum."Enabled", enum."Disabled and Grayed Out", enum."Enabled", enum."Disabled and Grayed Out"] items=["Enabled", "Disabled", "Disabled and Grayed Out"]  # 6.3.2, 6.3.3, 6.3.4
            }
            frame "6.3.6 온습도 싸이클 시험" {
              w120 = T7 [enum."Enabled", enum."Enabled", enum."Enabled", enum."Enabled", enum."Enabled", enum."Enabled", enum."Enabled", enum."Enabled", enum."Enabled", enum."Enabled", enum."Enabled", enum."Enabled", enum."Enabled", enum."Enabled", enum."Enabled", enum."Enabled", enum."Enabled", enum."Enabled", enum."Enabled", enum."Disabled and Grayed Out", enum."Enabled", enum."Enabled", enum."Disabled and Grayed Out", enum."Enabled", enum."Disabled and Grayed Out"] items=["Enabled", "Disabled", "Disabled and Grayed Out"]  # 6.3.6
            }
            frame "6.3.7 고온고습 방치" {
              w121 = T7 [enum."Enabled", enum."Enabled", enum."Enabled", enum."Disabled and Grayed Out", enum."Enabled", enum."Enabled", enum."Enabled", enum."Enabled", enum."Enabled", enum."Enabled", enum."Enabled", enum."Enabled", enum."Enabled", enum."Enabled", enum."Enabled", enum."Enabled", enum."Enabled", enum."Enabled", enum."Enabled", enum."Disabled and Grayed Out", enum."Enabled", enum."Disabled and Grayed Out", enum."Disabled and Grayed Out", enum."Enabled", enum."Enabled"] items=["Enabled", "Disabled", "Disabled and Grayed Out"]  # 6.3.8
            }
            frame "6.3.8 결로 시험" {
              w122 = T7 [enum."Enabled", enum."Enabled", enum."Enabled", enum."Disabled and Grayed Out", enum."Enabled", enum."Enabled", enum."Enabled", enum."Enabled", enum."Enabled", enum."Enabled", enum."Enabled", enum."Enabled", enum."Enabled", enum."Enabled", enum."Enabled", enum."Enabled", enum."Enabled", enum."Enabled", enum."Enabled", enum."Disabled and Grayed Out", enum."Enabled", enum."Enabled", enum."Enabled", enum."Enabled", enum."Enabled"] items=["Enabled", "Disabled", "Disabled and Grayed Out"]  # 6.3.8
            }
            frame "6.3.9 빙결시험" {
              w123 = T7 [enum."Enabled", enum."Enabled", enum."Enabled", enum."Disabled and Grayed Out", enum."Enabled", enum."Enabled", enum."Enabled", enum."Enabled", enum."Enabled", enum."Enabled", enum."Enabled", enum."Enabled", enum."Enabled", enum."Enabled", enum."Enabled", enum."Enabled", enum."Enabled", enum."Enabled", enum."Enabled", enum."Disabled and Grayed Out", enum."Enabled", enum."Enabled", enum."Disabled and Grayed Out", enum."Enabled", enum."Enabled"] items=["Enabled", "Disabled", "Disabled and Grayed Out"]  # 6.3.9
            }
            frame "6.3.10 공진" {
              w124 = T7 [enum."Enabled", enum."Enabled", enum."Enabled", enum."Enabled", enum."Disabled and Grayed Out", enum."Disabled and Grayed Out", enum."Enabled", enum."Enabled", enum."Enabled", enum."Enabled", enum."Enabled", enum."Enabled", enum."Enabled", enum."Enabled", enum."Enabled", enum."Enabled", enum."Enabled", enum."Enabled", enum."Enabled", enum."Disabled and Grayed Out", enum."Enabled", enum."Disabled and Grayed Out", enum."Disabled and Grayed Out", enum."Enabled", enum."Disabled and Grayed Out"] items=["Enabled", "Disabled", "Disabled and Grayed Out"]  # 동작시험
            }
            frame "6.3.11.1 작동가진" {
              w125 = T7 [enum."Enabled", enum."Enabled", enum."Enabled", enum."Enabled", enum."Disabled and Grayed Out", enum."Disabled and Grayed Out", enum."Enabled", enum."Enabled", enum."Enabled", enum."Enabled", enum."Enabled", enum."Enabled", enum."Enabled", enum."Enabled", enum."Enabled", enum."Enabled", enum."Enabled", enum."Enabled", enum."Enabled", enum."Disabled and Grayed Out", enum."Enabled", enum."Disabled and Grayed Out", enum."Disabled and Grayed Out", enum."Enabled", enum."Disabled and Grayed Out"] items=["Enabled", "Disabled", "Disabled and Grayed Out"]  # 동작시험
            }
            frame "6.3.11.2 비작동 가진 " {
              w126 = T7 [enum."Enabled", enum."Enabled", enum."Enabled", enum."Enabled", enum."Disabled and Grayed Out", enum."Disabled and Grayed Out", enum."Enabled", enum."Enabled", enum."Enabled", enum."Enabled", enum."Enabled", enum."Enabled", enum."Enabled", enum."Enabled", enum."Enabled", enum."Enabled", enum."Enabled", enum."Enabled", enum."Enabled", enum."Disabled and Grayed Out", enum."Enabled", enum."Disabled and Grayed Out", enum."Disabled and Grayed Out", enum."Enabled", enum."Disabled and Grayed Out"] items=["Enabled", "Disabled", "Disabled and Grayed Out"]  # 동작시험
            }
            frame "6.3.12 충격시험" {
              w127 = T7 [enum."Enabled", enum."Enabled", enum."Enabled", enum."Enabled", enum."Disabled and Grayed Out", enum."Disabled and Grayed Out", enum."Enabled", enum."Enabled", enum."Enabled", enum."Enabled", enum."Enabled", enum."Enabled", enum."Enabled", enum."Enabled", enum."Enabled", enum."Enabled", enum."Enabled", enum."Enabled", enum."Enabled", enum."Disabled and Grayed Out", enum."Enabled", enum."Disabled and Grayed Out", enum."Disabled and Grayed Out", enum."Enabled", enum."Disabled and Grayed Out"] items=["Enabled", "Disabled", "Disabled and Grayed Out"]  # 동작시험
            }
          }
          n34 = for {
            tunnel: w114 -> [w129] mode=indexing
            tunnel: w112 -> [w128] mode=indexing
            n35 = property class="Ctl"(reference=w129, "DisabledEnum"=w128) -> ()  [unwired: 1 in, 2 out]
          }
        }
        frame #2 {
          w135 = T7 [enum."Disabled and Grayed Out", enum."Disabled and Grayed Out", enum."Disabled and Grayed Out", enum."Enabled", enum."Disabled and Grayed Out", enum."Disabled and Grayed Out", enum."Disabled and Grayed Out", enum."Disabled and Grayed Out", enum."Enabled", enum."Disabled and Grayed Out"] items=["Enabled", "Disabled", "Disabled and Grayed Out"]
          n36 = case shown="True" w132 {
            tunnel: w134 -> [_ w141]
            tunnel: w133 -> [_ w140]
            tunnel: w131 -> [_ w139]
            tunnel: [_ w138] -> w130
            frame False {
            }
            frame True {
              n37 = Index Array(array=w139, index=w141) -> (element=w138:T1)
              n38 = property class="Clust (strict)"(reference=w140, "Value"=w138) -> ()  [unwired: 1 in, 2 out]
            }
          }
          n39 = property class="Clust (strict)"(reference=w137) -> ("Controls[]"=w136:refnum<vi>[])  [unwired: 1 in, 2 out]
          n40 = for {
            tunnel: w136 -> [w143] mode=indexing
            tunnel: w135 -> [w142] mode=indexing
            n41 = property class="Ctl"(reference=w143, "DisabledEnum"=w142) -> ()  [unwired: 1 in, 2 out]
          }
        }
      }
    }
    frame "고전압모드 동작검사" {
      n42 = stacked-sequence {
        seq-local: [w150 _ _] -> [_ w158 w178]
        tunnel: w149 -> [w151 w159 w177]
        tunnel: w148 -> [_ _ w182]
        tunnel: w147 -> [_ _ w179]
        tunnel: w146 -> [_ _ w176]
        tunnel: [_ _ w175] -> w145
        tunnel: w144 -> [w150 _ _]
        frame #0 {
          n43 = property class="Clust (strict)"(reference=w151) -> ("Controls[]"=w154:refnum<vi>[])  [unwired: 1 in, 2 out]
          n44 = Index Array(array=w154, index=0) -> (element=w155:refnum<vi>)
          n45 = property class="Ctl"(reference=w155) -> ("Value"=w153:variant)  [unwired: 1 in, 2 out]
          n46 = Variant To Data(type=T6."6.3.2 저온 작동/방치 시험" ("Test Mode"), Variant=w153) -> ()  [unwired: 1 in, 2 out]
        }
        frame #1 {
          n47 = property class="Clust (strict)"(reference=w159) -> ("Controls[]"=w160:refnum<vi>[])  [unwired: 1 in, 2 out]
          n48 = case shown="\"6.3.7 고온고습 방치\"" w158 {
            tunnel: [w161 w162 w163 w164 w165 w166 w167 w168 w169 w170 w171 w172] -> w157
            frame "6.3.1 온도방치 시험" {
              w161 = T7 [enum."Enabled", enum."Enabled", enum."Enabled", enum."Disabled and Grayed Out", enum."Enabled", enum."Enabled", enum."Enabled", enum."Enabled", enum."Enabled", enum."Enabled", enum."Enabled", enum."Enabled", enum."Enabled", enum."Enabled", enum."Enabled", enum."Enabled", enum."Enabled", enum."Enabled", enum."Enabled", enum."Enabled", enum."Enabled", enum."Disabled and Grayed Out", enum."Disabled and Grayed Out", enum."Enabled", enum."Enabled"] items=["Enabled", "Disabled", "Disabled and Grayed Out"]  # 6.3.8 (HV)
            }
            frame "6.3.2 저온 작동/방치 시험", Default {
              w162 = T7 [enum."Enabled", enum."Enabled", enum."Enabled", enum."Enabled", enum."Enabled", enum."Disabled and Grayed Out", enum."Enabled", enum."Enabled", enum."Enabled", enum."Enabled", enum."Enabled", enum."Enabled", enum."Enabled", enum."Enabled", enum."Enabled", enum."Enabled", enum."Enabled", enum."Enabled", enum."Enabled", enum."Enabled", enum."Enabled", enum."Enabled", enum."Disabled and Grayed Out", enum."Enabled", enum."Disabled and Grayed Out"] items=["Enabled", "Disabled", "Disabled and Grayed Out"]  # 6.3.2, 6.3.3, 6.3.4 (HV)
            }
            frame "6.3.3 고온 작동/방치 시험" {
              w163 = T7 [enum."Enabled", enum."Enabled", enum."Enabled", enum."Enabled", enum."Enabled", enum."Disabled and Grayed Out", enum."Enabled", enum."Enabled", enum."Enabled", enum."Enabled", enum."Enabled", enum."Enabled", enum."Enabled", enum."Enabled", enum."Enabled", enum."Enabled", enum."Enabled", enum."Enabled", enum."Enabled", enum."Enabled", enum."Enabled", enum."Enabled", enum."Disabled and Grayed Out", enum."Enabled", enum."Disabled and Grayed Out"] items=["Enabled", "Disabled", "Disabled and Grayed Out"]  # 6.3.2, 6.3.3, 6.3.4 (HV)
            }
            frame "6.3.4 온도 싸이클 시험" {
              w164 = T7 [enum."Enabled", enum."Enabled", enum."Enabled", enum."Enabled", enum."Enabled", enum."Disabled and Grayed Out", enum."Enabled", enum."Enabled", enum."Enabled", enum."Enabled", enum."Enabled", enum."Enabled", enum."Enabled", enum."Enabled", enum."Enabled", enum."Enabled", enum."Enabled", enum."Enabled", enum."Enabled", enum."Enabled", enum."Enabled", enum."Enabled", enum."Disabled and Grayed Out", enum."Enabled", enum."Disabled and Grayed Out"] items=["Enabled", "Disabled", "Disabled and Grayed Out"]  # 6.3.2, 6.3.3, 6.3.4 (HV)
            }
            frame "6.3.6 온습도 싸이클 시험" {
              w165 = T7 [enum."Enabled", enum."Enabled", enum."Enabled", enum."Enabled", enum."Enabled", enum."Enabled", enum."Enabled", enum."Enabled", enum."Enabled", enum."Enabled", enum."Enabled", enum."Enabled", enum."Enabled", enum."Enabled", enum."Enabled", enum."Enabled", enum."Enabled", enum."Enabled", enum."Enabled", enum."Enabled", enum."Enabled", enum."Enabled", enum."Disabled and Grayed Out", enum."Enabled", enum."Disabled and Grayed Out"] items=["Enabled", "Disabled", "Disabled and Grayed Out"]  # 6.3.6 (HV)
            }
            frame "6.3.7 고온고습 방치" {
              w166 = T7 [enum."Enabled", enum."Enabled", enum."Enabled", enum."Disabled and Grayed Out", enum."Enabled", enum."Enabled", enum."Enabled", enum."Enabled", enum."Enabled", enum."Enabled", enum."Enabled", enum."Enabled", enum."Enabled", enum."Enabled", enum."Enabled", enum."Enabled", enum."Enabled", enum."Enabled", enum."Enabled", enum."Enabled", enum."Enabled", enum."Disabled and Grayed Out", enum."Disabled and Grayed Out", enum."Enabled", enum."Enabled"] items=["Enabled", "Disabled", "Disabled and Grayed Out"]  # 6.3.8 (HV)
            }
            frame "6.3.8 결로 시험" {
              w167 = T7 [enum."Enabled", enum."Enabled", enum."Enabled", enum."Disabled and Grayed Out", enum."Enabled", enum."Enabled", enum."Enabled", enum."Enabled", enum."Enabled", enum."Enabled", enum."Enabled", enum."Enabled", enum."Enabled", enum."Enabled", enum."Enabled", enum."Enabled", enum."Enabled", enum."Enabled", enum."Enabled", enum."Enabled", enum."Enabled", enum."Enabled", enum."Enabled", enum."Enabled", enum."Enabled"] items=["Enabled", "Disabled", "Disabled and Grayed Out"]  # 6.3.8 (HV)
            }
            frame "6.3.9 빙결시험" {
              w168 = T7 [enum."Enabled", enum."Enabled", enum."Enabled", enum."Disabled and Grayed Out", enum."Enabled", enum."Enabled", enum."Enabled", enum."Enabled", enum."Enabled", enum."Enabled", enum."Enabled", enum."Enabled", enum."Enabled", enum."Enabled", enum."Enabled", enum."Enabled", enum."Enabled", enum."Enabled", enum."Enabled", enum."Enabled", enum."Enabled", enum."Enabled", enum."Disabled and Grayed Out", enum."Enabled", enum."Enabled"] items=["Enabled", "Disabled", "Disabled and Grayed Out"]  # 6.3.9 (HV)
            }
            frame "6.3.10 공진" {
              w169 = T7 [enum."Enabled", enum."Enabled", enum."Enabled", enum."Enabled", enum."Disabled and Grayed Out", enum."Disabled and Grayed Out", enum."Enabled", enum."Enabled", enum."Enabled", enum."Enabled", enum."Enabled", enum."Enabled", enum."Enabled", enum."Enabled", enum."Enabled", enum."Enabled", enum."Enabled", enum."Enabled", enum."Enabled", enum."Disabled and Grayed Out", enum."Enabled", enum."Disabled and Grayed Out", enum."Disabled and Grayed Out", enum."Enabled", enum."Disabled and Grayed Out"] items=["Enabled", "Disabled", "Disabled and Grayed Out"]  # 동작시험
            }
            frame "6.3.11.1 작동가진" {
              w170 = T7 [enum."Enabled", enum."Enabled", enum."Enabled", enum."Enabled", enum."Disabled and Grayed Out", enum."Disabled and Grayed Out", enum."Enabled", enum."Enabled", enum."Enabled", enum."Enabled", enum."Enabled", enum."Enabled", enum."Enabled", enum."Enabled", enum."Enabled", enum."Enabled", enum."Enabled", enum."Enabled", enum."Enabled", enum."Disabled and Grayed Out", enum."Enabled", enum."Disabled and Grayed Out", enum."Disabled and Grayed Out", enum."Enabled", enum."Disabled and Grayed Out"] items=["Enabled", "Disabled", "Disabled and Grayed Out"]  # 동작시험
            }
            frame "6.3.11.2 비작동 가진 " {
              w171 = T7 [enum."Enabled", enum."Enabled", enum."Enabled", enum."Enabled", enum."Disabled and Grayed Out", enum."Disabled and Grayed Out", enum."Enabled", enum."Enabled", enum."Enabled", enum."Enabled", enum."Enabled", enum."Enabled", enum."Enabled", enum."Enabled", enum."Enabled", enum."Enabled", enum."Enabled", enum."Enabled", enum."Enabled", enum."Disabled and Grayed Out", enum."Enabled", enum."Disabled and Grayed Out", enum."Disabled and Grayed Out", enum."Enabled", enum."Disabled and Grayed Out"] items=["Enabled", "Disabled", "Disabled and Grayed Out"]  # 동작시험
            }
            frame "6.3.12 충격시험" {
              w172 = T7 [enum."Enabled", enum."Enabled", enum."Enabled", enum."Enabled", enum."Disabled and Grayed Out", enum."Disabled and Grayed Out", enum."Enabled", enum."Enabled", enum."Enabled", enum."Enabled", enum."Enabled", enum."Enabled", enum."Enabled", enum."Enabled", enum."Enabled", enum."Enabled", enum."Enabled", enum."Enabled", enum."Enabled", enum."Disabled and Grayed Out", enum."Enabled", enum."Disabled and Grayed Out", enum."Disabled and Grayed Out", enum."Enabled", enum."Disabled and Grayed Out"] items=["Enabled", "Disabled", "Disabled and Grayed Out"]  # 동작시험
            }
          }
          n49 = for {
            tunnel: w160 -> [w174] mode=indexing
            tunnel: w157 -> [w173] mode=indexing
            n50 = property class="Ctl"(reference=w174, "DisabledEnum"=w173) -> ()  [unwired: 1 in, 2 out]
          }
        }
        frame #2 {
          w180 = T7 [enum."Enabled", enum."Enabled", enum."Enabled", enum."Enabled", enum."Enabled", enum."Enabled", enum."Enabled", enum."Enabled", enum."Enabled", enum."Enabled"] items=["Enabled", "Disabled", "Disabled and Grayed Out"]
          n51 = case shown="True" w176 {
            tunnel: w179 -> [_ w186]
            tunnel: w178 -> [_ w185]
            tunnel: w177 -> [_ w184]
            tunnel: [_ w183] -> w175
            frame False {
            }
            frame True {
              n52 = Index Array(array=w186, index=w185) -> (element=w183:T1)
              n53 = property class="Clust (strict)"(reference=w184, "Value"=w183) -> ()  [unwired: 1 in, 2 out]
            }
          }
          n54 = property class="Clust (strict)"(reference=w182) -> ("Controls[]"=w181:refnum<vi>[])  [unwired: 1 in, 2 out]
          n55 = for {
            tunnel: w181 -> [w188] mode=indexing
            tunnel: w180 -> [w187] mode=indexing
            n56 = property class="Ctl"(reference=w188, "DisabledEnum"=w187) -> ()  [unwired: 1 in, 2 out]
          }
        }
      }
    }
  }
  "conf'" <- w39
  "error out" <- "error in (no error)"
